vi "Confirm Sub-Block.vi"(8 "error in":errorcluster, 11 "Block Upload Transfer in":refnum<class "Block Upload Sub-Block Transfer.lvclass">) -> (0 "error out":errorcluster, 3 "Block Upload Transfer out":refnum<class "Block Upload Sub-Block Transfer.lvclass">)   [LabVIEW 2020, in "CANopen.lvlib" / "SDO Manager.lvlib" / "Block Upload Sub-Block Transfer.lvclass"]
uses:
  Block Upload Sub-Block Transfer.lvclass
  Block Upload Sub-Block Transfer.lvclass/Block Upload Sub-Block Transfer.ctl
  HAL/Source/Interfaces/ICommunicate/ICommunicate.lvclass
  CANopen Message/CANopen Message.lvclass
  Typedefs/Function Code.ctl
  CANopen.lvlib
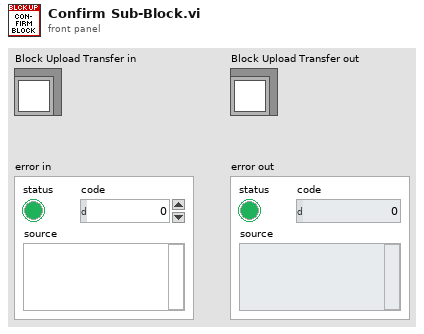
[diagram p1: front panel]
types:
  T1 = typedef "CANopen.lvlib/Function Code.ctl" = u8
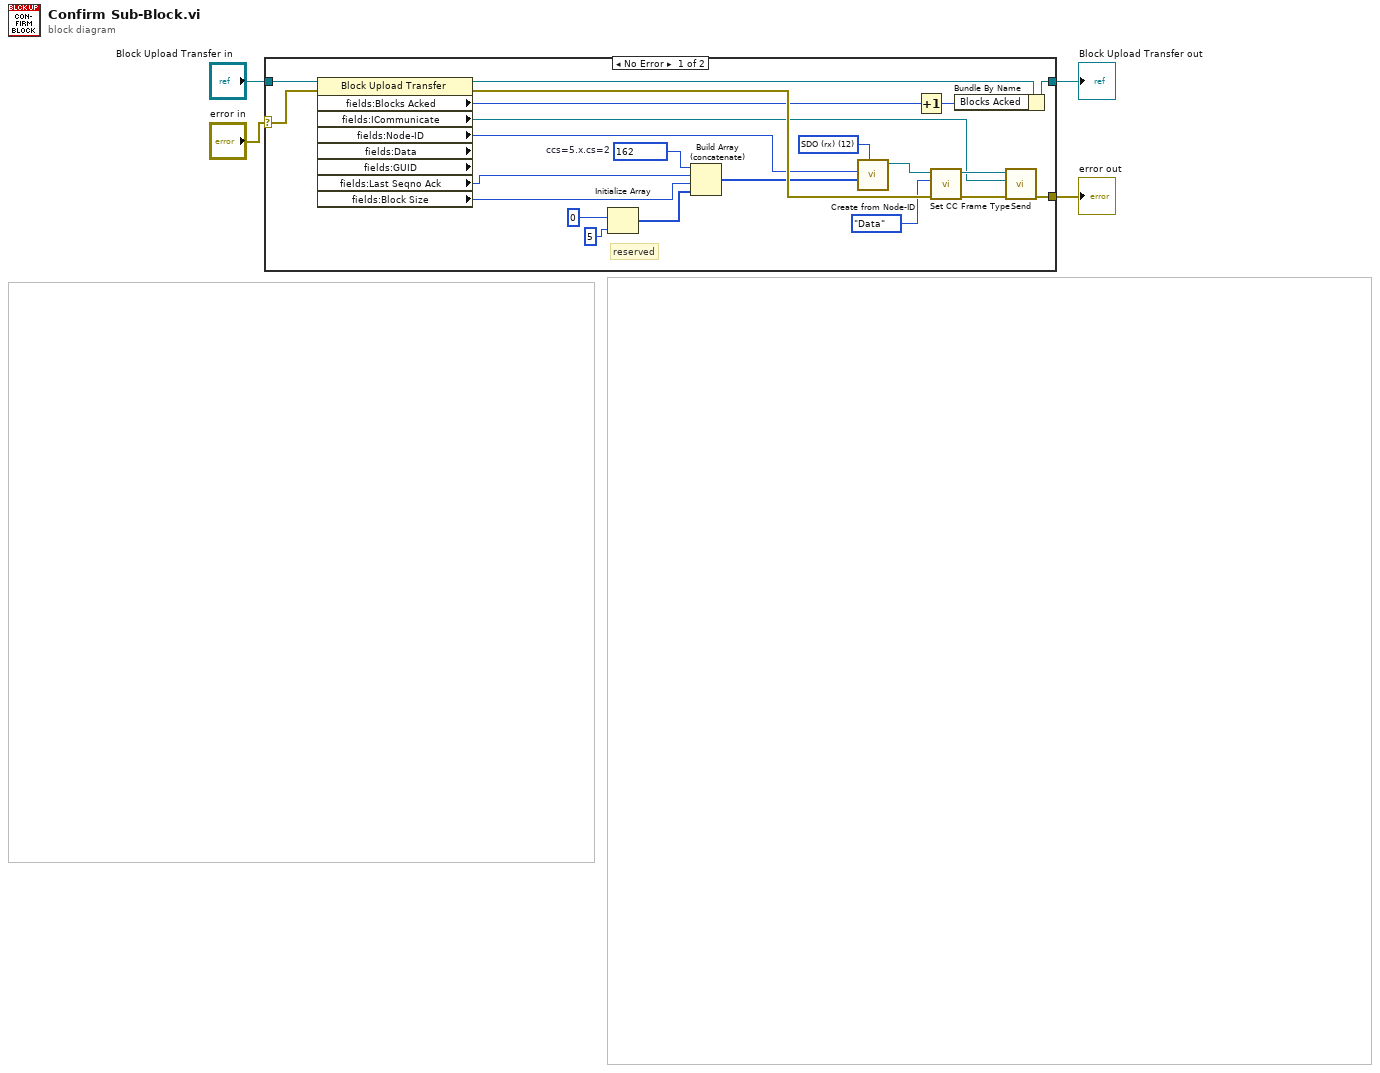
[diagram p0: block diagram]
diagram:
  n1 = case shown="No Error" "error in" {
    selector: "error in" -> [w25 w27]
    tunnel: "Block Upload Transfer in" -> [w24 w28]
    tunnel: [w7 w28] -> w1
    tunnel: [w22 w27] -> w2
    frame No Error {
      w17 = T1 12 items=["NMT"=0, "EMCY/SYNC"=1, "TIME"=2, "PDO1 (tx)"=3, "PDO1 (rx)"=4, "PDO2 (tx)"=5, "PDO2 (rx)"=6, "PDO3 (tx)"=7, "PDO3 (rx)"=8, "PDO4 (tx)"=9, "PDO4 (rx)"=10, "SDO (tx)"=11, "SDO (rx)"=12, "NMT error control"=14] ("Function Code")
      w20 = u8 162  # ccs=5.x.cs=2
      # "reserved"
      n2 = property class="Block Upload Transfer" props=["fields:Blocks Acked", "fields:ICommunicate", "fields:Node-ID", "fields:Data", "fields:GUID", "fields:Last Seqno Ack", "fields:Block Size"](reference=w24, error in=w25) -> (reference out=w23:refnum<class "Block Upload Sub-Block Transfer.lvclass">, error out=w26:errorcluster, "fields:Blocks Acked"=w5:u8, "fields:ICommunicate"=w8:refnum<class "ICommunicate.lvclass">, "fields:Node-ID"=w21:u8, "fields:Last Seqno Ack"=w12:u8, "fields:Block Size"=w11:u8)  [unwired: 2 out]
      n3 = Initialize Array(u8 0, 5 ("y")) -> (w10:u8[])
      n4 = Build Array (concatenate)(w20, w12, w11, w10) -> (w18:u8[])
      n5 = call "Create from Node-ID.vi"("Function Code"=w17, "Data"=w18, "Node-ID"=w21) -> ("CANopen Message"=w16:refnum<class "CANopen Message.lvclass">)  [unwired: 8 in]
      n6 = Increment(x=w5) -> (x+1=w6:u8)
      n7 = call "Set CC Frame Type.vi"("error in"=w26, "CC Frame Type"=enum8{"Data", "Remote", "Error", "Overload"}."Data", "CANopen Message in"=w16) -> ("error out"=w15:errorcluster, "CANopen Message out"=w14:refnum<class "CANopen Message.lvclass">)  [unwired: 7 in]
      n8 = Bundle By Name(cluster=w23, "Blocks Acked"=w6) -> (w7:refnum<class "Block Upload Sub-Block Transfer.lvclass">)
      n9 = call "Send.vi"("error in"=w15, "ICommunicate"=w8, "CANopen Message in"=w14) -> ("error out"=w22:errorcluster)  [unwired: 7 in, 1 out]
    }
    frame Error {
    }
  }
  "Block Upload Transfer out" <- w1
  "error out" <- w2
